vi "TDOanalysis.vi"() -> ()   [LabVIEW 2021]
uses:
  ark_all/arkady-arxiv/oldTDOanalysis/Data window.ctl
  ark_all/arkady-arxiv/agregator -- action.ctl
  ark_all/arkady-arxiv/interpolation state - real.ctl
  ark_all/arkady-arxiv/filename-action.ctl
  <vilib>/Analysis/4window.llb/Hanning Window (DBL).vi
  <vilib>/Analysis/4window.llb/Blackman Window (DBL).vi
  <vilib>/Analysis/baseanly.llb/Mean (DBL).vi
  <vilib>/Analysis/8numeric.llb/1D Numeric Integration.vi
  ark_all/arkady-arxiv/linear interpolation - real -- V2.vi
  <vilib>/Analysis/4window.llb/AllCosWindow (DBL).vi
  <vilib>/Analysis/baseanly.llb/A x B.vi
  <vilib>/Analysis/baseanly.llb/Real A x B.vi
  ark_all/arkady-arxiv/Q -- check range -- i -- real.vi
  ark_all/arkady-arxiv/line -- complex.vi
  ark_all/arkady-arxiv/Q -- check range -- i -- integer.vi
  ark_all/arkady-arxiv/Q - not nan -- real.vi
  ark_all/arkady-arxiv/Q - not nan -- integer.vi
  <vilib>/measure/matone.llb/Extract Single Tone Information 1 Chan.vi
  <vilib>/Waveform/WDTOps.llb/WDT Number of Waveform Samples DBL.vi
  <vilib>/Analysis/Matrix/Numeric/Conversions/Array To Matrix.vi
  <vilib>/Analysis/Matrix/Numeric/Conversions/Array To Matrix - RA2.vi
  <vilib>/Analysis/baseanly.llb/Inverse Matrix.vi
  <vilib>/Analysis/baseanly.llb/Real Inverse Matrix.vi
  <vilib>/Utility/file.llb/Write Delimited Spreadsheet (string).vi
  <vilib>/Utility/file.llb/Write Delimited Spreadsheet (DBL).vi
  <vilib>/Analysis/NI_AALPro.lvlib
  <vilib>/measure/NI_MAPro.lvlib
  <vilib>/Analysis/NI_AALBase.lvlib
  <vilib>/Analysis/NI_AAL_SigProc.lvlib
panel:
  in  "Tab Control":enum32{"Page 1", "Page 2", "Page 3"}(tab)
  in  "gamma window (sec)":dbl=0.0001 format="%#_6p"
  out "Gamma vs. Field":cluster{dbl[], dbl[]}(graph)
  out "Apmlitude or Pwr. vs. Field":cluster{dbl[], dbl[]}(graph)
  out "Frequency vs. Field":cluster{dbl[], dbl[]}(graph)
  out "Frequency vs. time":waveform(dbl)(graph)={"t0"=timestamp(-0.00999989999999995 s since 1904-01-01), "dt"=2e-05, "Y"=array[6499 elements]}
  out "Progress":dbl(slide)=1.0018766168281668 scale=0.0..1.0
  out "first line":string[](array[string])=["003_041224_time 003_041224_field 003_041224_freq 003_041224_amp 003_041224_gamma "]
  in  "remove file prefix":string="p_c3_"
  in  "?":enum32{"TDO Analysis Settings", "Page 2"}(tab)
  in  "Power spctr. threshold":dbl=0.0001 format="%.4f"
  in  "Freq. threshold":dbl=30000.0
  in  "window width (s)":dbl=0.0003 format="%#_6p"
  in  "window step (s)":dbl=2e-05 format="%#_6p"
  in  "detection method":T1(ring)
  in  "fit width":i32=9 min=3
  in  "window type":enum16{"Hanning", "Box", "Blackman"}(ring)
  in  "Input File":path=path "/Users/arkadyshekhter/Library/CloudStorage/Dropbox/shared_KimValBra/Apr2024— UTe2/041224/p_c3_003_041224.tdms"
  out "Ampl vs. time":waveform(dbl)(graph)={"t0"=timestamp(-0.00999989999999995 s since 1904-01-01), "dt"=2e-05, "Y"=array[6499 elements]}
  in  "add file suffix":string="_tdo_"
  in  "ovewrite file?":bool=TRUE
  in  "?":enum32{"data settings", "Field  Settings"}(tab)
  in  "Data channels (1st - Field, 2nd - TDO)":T2={"Start"=0, "Length"=10000, "Other frmt channel numbers"=[0], "TDMS Channel names"=["Field", "Vpick"], "TDMS Group name"="p"}
  in  "Data File Type":T3(ring)
  in  "Bdot Calibration Factor":dbl=3794.0
  out "B dot offset":dbl=-3.6804060216009077e-06 format="%.6f"
  in  "Length for Bdot offset, s":dbl=0.009 format="%#_6p"
  in  "Input field format":enum16{"Bdot", "B"}(ring)=enum."B"
  in  "Field correction":dbl=1.0
  out "Array":bool[](array[boolean])
  in  "upper limit":dbl
  in  "lower limit":dbl
  in  "Low-pass filter":T4={"Clip IIR filter ramps, in 1/Tc units"=1.0, "Two-pass & flip"=TRUE, "IIR filter specifications"={"Topology"=enum."Off", "Type"=enum."Lowpass", "Order"=1, "Lower Fc"=1e-06, "Upper Fc"=0.0, "PB Ripple"=1.0, "SB Attenuation"=60.0}} {"IIR filter specifications"."PB Ripple" format="%0.2f"; "IIR filter specifications"."Lower Fc" format="%0.2p"; "IIR filter specifications"."SB Attenuation" format="%0.2f"; "IIR filter specifications"."Upper Fc" format="%0.2p"}
  in  "error in":errorcluster
  out "Amplitude vs. Field (PWR peak)":cluster{dbl[], "Filtered X":dbl[]}(graph)
  out "size(s)":i32=6499
  in  "# of threads":i32=4
  out "Field profile":waveform(dbl)(graph)={"t0"=timestamp(-0.00999989999999995 s since 1904-01-01), "dt"=2e-05, "Y"=array[6468 elements]}
  in  "End, s":dbl=nan format="%.6f"
  in  "Start, s":dbl=nan format="%.6f"
  # "Basic NHMFL TDO routine\nv. 0.5       F. F. Balakirev\n\nmessed with by Arkady!"
  # "Background file is either an ASCII *.dat file produced by TDO earlier\nor *.fit file containing single column of polynomial fit coeficients.\n1st row in fit file is a text header, which is ingnored. Result is saved in a \n\"*diff.dat\" file in the output folder\nExample \"PDO1.fit\": \n\nFit y=A_i*x^i, starting with A_0\n3.25637E7\n2132.56863\n-12.60591\n-2.01013\n-0.04452\n-3.23119E-4"
  # "OR"
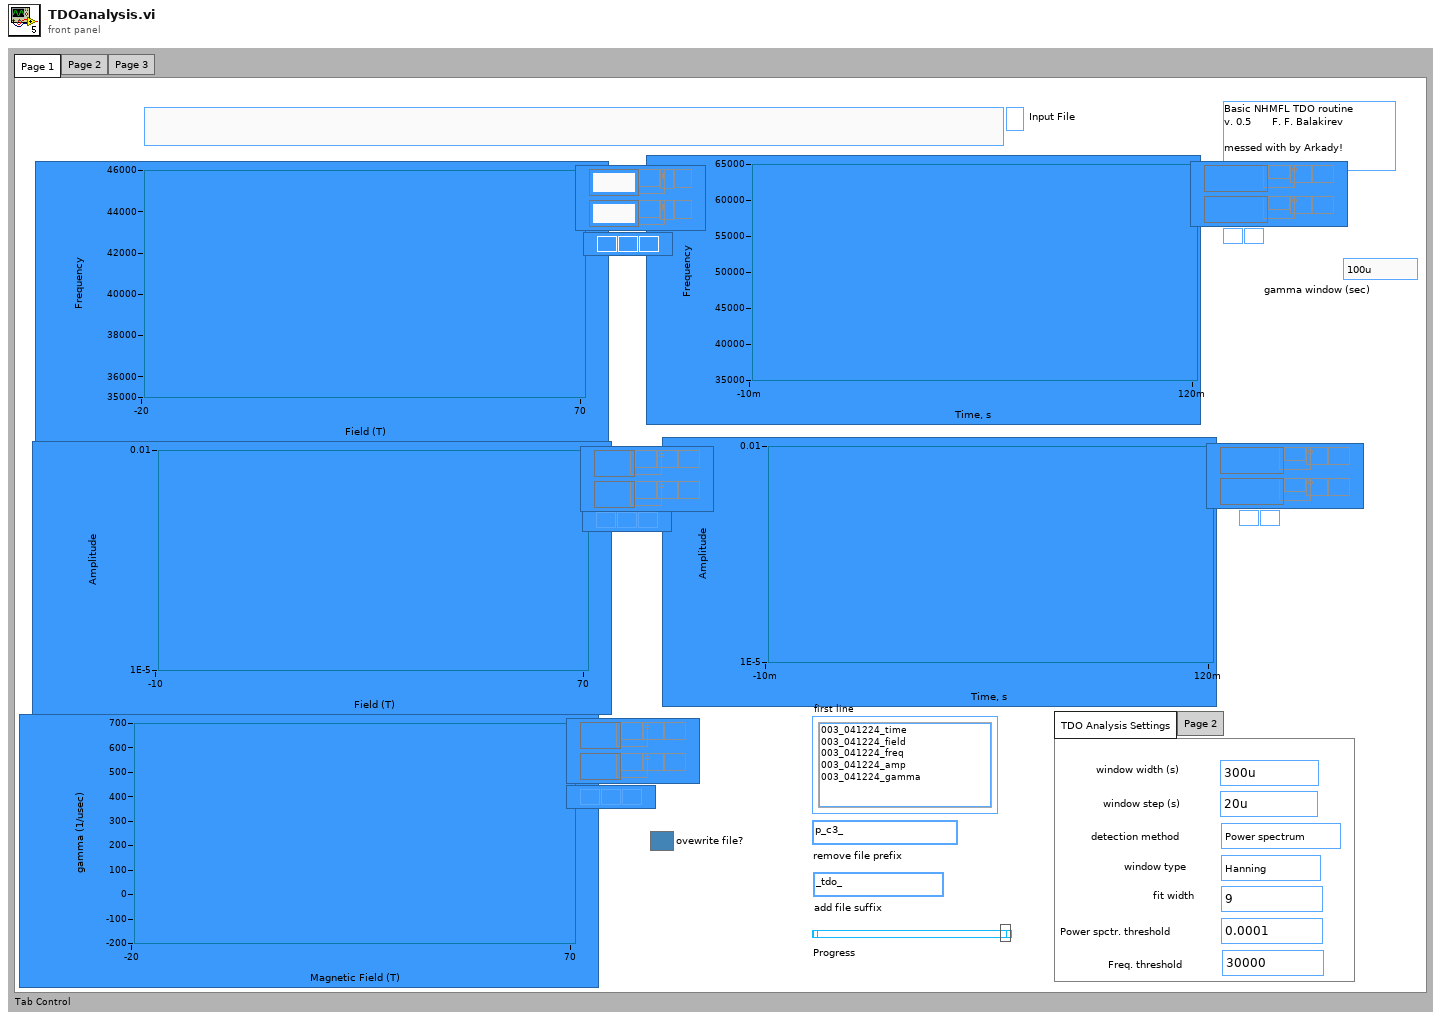
[diagram p1: front panel]
types:
  T1 = enum16{"Power spectrum", "Tone detection", "Peak-to-peak fit"}
  T2 = cluster{"Start":i64, "Length":i32, "Other frmt channel numbers":i64[], "TDMS Channel names":string[], "TDMS Group name":string}
  T3 = enum16{"TDMS file", "Tektronics ISF", "BinF file", "ASCII File", "BinH File", "BinW File", "BINARY File"}
  T4 = cluster{"Clip IIR filter ramps, in 1/Tc units":dbl, "Two-pass & flip":bool, "IIR filter specifications":cluster{"Topology":enum16{"Off", "Butterworth", "Chebyshev", "Inverse Chebyshev", "Elliptic", "Bessel"}, "Type":enum16{"Lowpass", "Highpass", "Bandpass", "Bandstop"}, "Order":i32, "Lower Fc":dbl, "Upper Fc":dbl, "PB Ripple":dbl, "SB Attenuation":dbl}}
  T5 = typedef "filename-action.ctl" = enum16{"rewrite", "parse", "force pattern", "uniquenum", "get T", "get B", "get ind", "get deg", "get name", "get folder", "get extension", "get basename", "get side", "get setof", "getID", "getIDStock", "remove prefix"}
  T6 = typedef "interpolation state - real.ctl" = cluster{"Array ":dbl[], "actual size":i32, "requested size":i32}
  T7 = typedef "agregator -- action.ctl" = enum16{"append", "interpolate", "empty!", "force", "init", "scale", "read last"}
  T8 = enum16{"Off", "Butterworth", "Chebyshev", "Inverse Chebyshev", "Elliptic", "Bessel"}
  T9 = cluster{"Start":i64, "Length":i64, "Channel numbers":i64[], "Channel names":string[], "Group name":string}
  T10 = typedef "Data window.ctl" = cluster{"Start":i64, "Length":i64, "Channel numbers":i64[], "Channel name":string, "Group name":string}
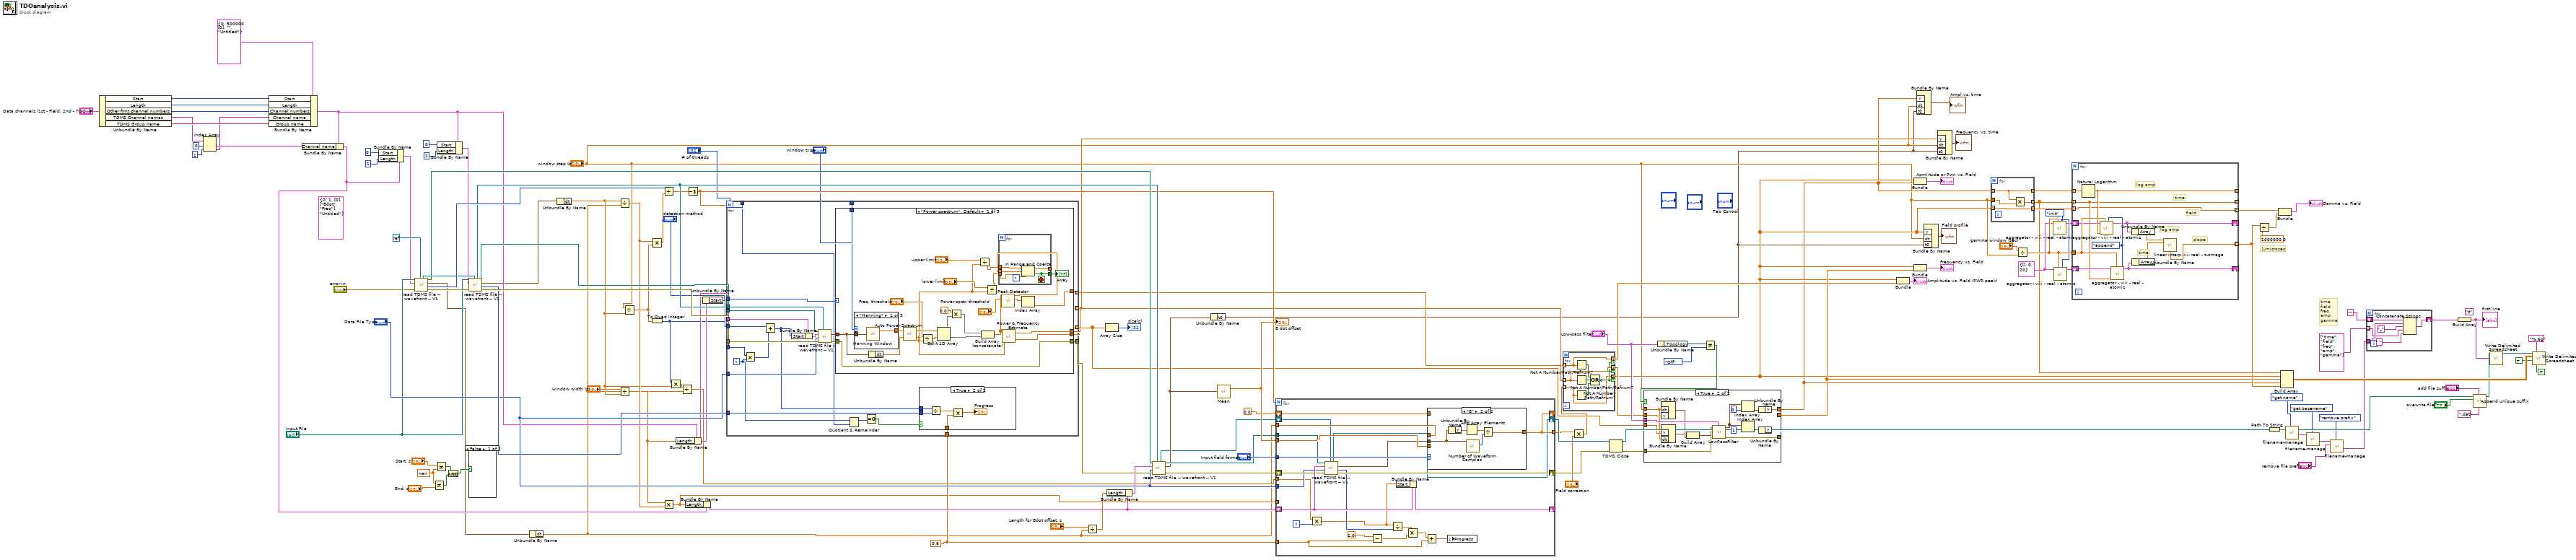
[diagram p0: block diagram]
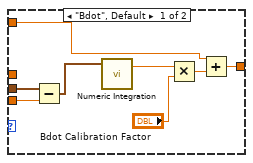
[diagram p2: hidden frame]
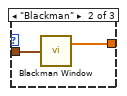
[diagram p5: hidden frame]
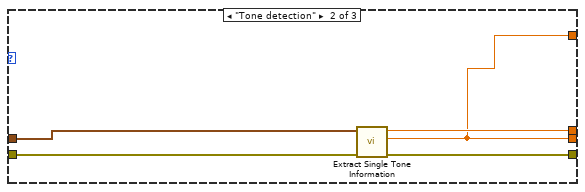
[diagram p7: hidden frame]
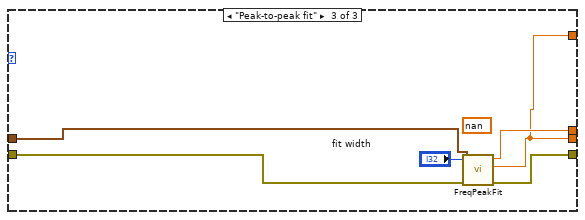
[diagram p8: hidden frame]
diagram:
  (unwired) "\t"
  w33 = T6 {"Array "=[], "actual size"=0, "requested size"=20} ("state IN")
  w38 = agregator_--_action."init" ("aggregator action")
  w68 = 0.6 ("y")
  (unwired) T9 {"Start"=0, "Length"=1, "Channel numbers"=[0], "Channel names"=["Bdot", "Freq"], "Group name"="Untitled"} ("Data window")
  w112 = nan
  # "1/microsec"
  # "time \nfield\nfreq\namp\ngamma"
  n1 = Unbundle By Name("Data channels (1st - Field, 2nd - TDO)") -> ("Start"=w118:i64, "Length"=w121:i32, "Other frmt channel numbers"=w120:i64[], "TDMS Channel names"=w100:string[], "TDMS Group name"=w119:string)
  n2 = Index Array(array=w100, index #1=0 ("index"), index #2=1 ("index")) -> (element #1=w117:string, element #2=w104:string)
  n3 = Bundle By Name(cluster=T10 {"Start"=0, "Length"=500000, "Channel numbers"=[0], "Channel name"="", "Group name"="Untitled"} ("Data window"), "Start"=w118, "Length"=w121, "Channel numbers"=w120, "Channel name"=w104, "Group name"=w119) -> (w102:T10)
  n4 = Bundle By Name(cluster=w102, "Channel name"=w117) -> (w116:T10)
  n5 = Bundle By Name(cluster=w116, "Start"=i64 0, "Length"=i64 1) -> (w97:T10)
  n6 = call "read TDMS file -- wavefront -- V1.vi"("tdms file in"=refnum<k0> refnum, "error in"="error in", "Data window"=w97, "Input file path"="Input File") -> ("error out"=w132:errorcluster, "1st channel length"=w126:u64, "Data out"=w99:waveform(dbl), "Actual input file path"=w128:path, "tdms file out"=w106:refnum<k34>)  [unwired: 3 in]
  n7 = Not Equal?(x=w112, y="End, s") -> (x != y?=w109:bool)
  n8 = Not Equal?(x="Start, s", y=w112) -> (x != y?=w110:bool)
  n9 = Bundle By Name(cluster=w102, "Start"=i64 0, "Length"=i64 1) -> (w96:T10)
  n10 = And(x=w110, y=w109) -> (x .and. y?=w108:bool)
  n11 = case shown="False" w108 {
    frame False {
    }
    frame True {
    }
  }
  n12 = call "read TDMS file -- wavefront -- V1.vi"("tdms file in"=w106, "error in"=w132, "Data window"=w96, "Input file path"="Input File") -> ("error out"=w129:errorcluster, "1st channel length"=w125:u64, "Data out"=w98:waveform(dbl), "Actual input file path"=w131:path, "tdms file out"=w107:refnum<k34>)  [unwired: 3 in]
  n13 = Unbundle By Name(w99) -> ("dt"=w31:dbl)
  n14 = Unbundle By Name(w98) -> ("dt"=w32:dbl)
  n15 = Divide(x=w32, y=w31) -> (x/y=w62:dbl)
  n16 = Divide(x="window width (s)", y=w32) -> (x/y=w57:dbl)
  n17 = Divide(x="window step (s)", y=w32) -> (x/y=w88:dbl)
  n18 = Multiply(x=w62, y=w88) -> (x*y=w76:dbl)
  n19 = To Quad Integer(1:w88) -> (0:w56:i64)
  n20 = Divide(x=w126, y=w76) -> (x/y=w95:dbl)
  n21 = Multiply(x=w57, y=w62) -> (x*y=w58:dbl)
  n22 = Multiply(x=w56, y=w32) -> (x*y=w55:dbl)
  n23 = Bundle By Name(cluster=w102, "Length"=w57) -> (w61:T10)
  n24 = Divide(x=w55, y=w31) -> (x/y=w54:dbl)
  n25 = Bundle By Name(cluster=w116, "Length"=w58) -> (w77:T10)
  n26 = Decrement(x=w95) -> (x-1=w69:dbl)
  n27 = Unbundle By Name(w61) -> ("Start"=w60:i64)
  n28 = for {
    N: w69 -> [_]
    tunnel: [w152] -> w51 mode=indexing
    tunnel: [w157] -> w52 mode=indexing
    tunnel: [w156] -> w50 mode=indexing
    tunnel: "Data File Type" -> [w153]
    tunnel: w131 -> [w154]
    tunnel: w56 -> [w145]
    tunnel: "detection method" -> [w151]
    tunnel: w125 -> [w150]
    tunnel: w68 -> [w147]
    tunnel: w61 -> [w144]
    tunnel: w60 -> [w143]
    tunnel: w129 -> [w155]
    tunnel: [w149] -> w71
    tunnel: "window type" -> [w141]
    tunnel: w107 -> [w135]
    tunnel: "# of threads" -> [w134]
    i -> [w138]
    n29 = Multiply(x=w145, y=w138) -> (x*y=w139:i64)
    n30 = Add(x=w143, y=w139) -> (x+y=w140:i64)
    n31 = Bundle By Name(cluster=w144, "Start"=w140) -> (w142:T10)
    n32 = call "read TDMS file -- wavefront -- V1.vi"("tdms file in"=w135, "error in"=w155, "Data File Type"=w153, "Data window"=w142, "Input file path"=w154) -> ("error out"=w148:errorcluster, "Data out"=w146:waveform(dbl))  [unwired: 2 in, 3 out]
    n33 = case shown="\"Power spectrum\", Default" w151 {
      tunnel: [w186 w198 w203] -> w157
      tunnel: [w167 w198 w203] -> w156
      tunnel: w146 -> [w185 w201 w208]
      tunnel: [w174 w202 w207] -> w152
      tunnel: w148 -> [w176 w200 w205]
      tunnel: [w176 w199 w204] -> w149
      tunnel: w141 -> [w175 _ _]
      frame "Power spectrum", Default {
        n34 = case shown="\"Hanning\"" w175 {
          tunnel: [w194 w196 w197] -> w187
          tunnel: w185 -> [w193 w195 w197]
          frame "Hanning" {
            n35 = call-poly <vilib>:"Hanning Window.vi"("X"=w193) -> ("Windowed X"=w194:dbl[])  [unwired: 1 out]
          }
          frame "Blackman" {
            n36 = call-poly <vilib>:"Blackman Window.vi"("X"=w195) -> ("Windowed X"=w196:dbl[])  [unwired: 1 out]
          }
          frame "Box" {
          }
        }
        n37 = Unbundle By Name(w185) -> ("dt"=w184:dbl)
        n38 = call <vilib>:"Auto Power Spectrum.vi"("dt"=w184, "Signal (V)"=w187) -> ("df"=w171:dbl, "Power Spectrum (V^2 rms)"=w182:dbl[])
        n39 = Divide(x="Freq. threshold", y=w171) -> (x/y=w181:dbl)
        n40 = Split 1D Array(array=w182, index=w181) -> (first subarray=w178:dbl[], second subarray=w180:dbl[])
        n41 = Multiply(x=0.0 ("element"), y=w178) -> (x*y=w177:dbl[])
        n42 = Divide(x="upper limit", y=w171) -> (x/y=w169:dbl)
        n43 = Build Array (concatenate)(w177, w180) -> (w166:dbl[])
        n44 = Divide(x="lower limit", y=w171) -> (x/y=w172:dbl)
        n45 = call <vilib>:"Peak Detector.vi"("threshold"="Power spctr. threshold", "X"=w166) -> ("Amplitudes"=w163:dbl[], "Locations"=w164:dbl[])  [unwired: 5 in, 3 out]
        n46 = for {
          tunnel: w164 -> [w192] mode=indexing
          tunnel: w169 -> [w191]
          tunnel: w172 -> [w190]
          tunnel: [w189] -> _
          tunnel: [w188] -> w168 mode=indexing
          stop <- w188 stop-if-true
          n47 = In Range and Coerce(upper limit=w191, x=w192, lower limit=w190) -> (coerced(x)=w189:dbl, In Range?=w188:bool)
        }
        "Array" <- w168
        n48 = call <vilib>:"Power & Frequency Estimate.vi"("df"=w171, "Power Spectrum (V^2 rms)"=w166) -> ("est power peak"=w186:dbl, "est frequency peak"=w174:dbl)  [unwired: 3 in, 1 out]
        n49 = Index Array(array=w163) -> (element=w167:dbl)  [unwired: 1 in]
      }
      frame "Tone detection" {
        n50 = call-poly <vilib>:"Extract Single Tone Information.vi"("error in (no error)"=w200, "time signal in"=w201) -> ("error out"=w199:errorcluster, "detected amplitude"=w198:dbl, "detected frequency"=w202:dbl)  [unwired: 2 in, 5 out]
      }
      frame "Peak-to-peak fit" {
        (unwired) nan
        n51 = call "FreqPeakFit.vi"("error in (no error)"=w205, "Peak fit width"="fit width", "Waveform"=w208) -> ("error out"=w204:errorcluster, "Amplitude"=w203:dbl, "PeakFreqOut"=w207:dbl)  [unwired: 4 out]
      }
    }
    n52 = Quotient & Remainder(x=w138, y=w134) -> (x-y*floor(x/y)=w137:i32)  [unwired: 1 out]
    n53 = Equal To 0?(x=w137) -> (x = 0?=w136:bool)
    n54 = case shown="True" w136 {
      tunnel: w150 -> [_ w162]
      tunnel: w147 -> [_ w159]
      tunnel: w140 -> [_ w158]
      frame False {
      }
      frame True {
        n55 = Divide(x=w158, y=w162) -> (x/y=w161:dbl)
        n56 = Multiply(x=w161, y=w159) -> (x*y=→"Progress":dbl)
      }
    }
  }
  n57 = Divide(x="Length for Bdot offset, s", y=w31) -> (x/y=w79:dbl)
  n58 = Array Size(array=w52) -> (size(s)=→"size(s)":i32)
  n59 = Bundle By Name(cluster=w77, "Length"=w79) -> (w67:T10)
  n60 = call "read TDMS file -- wavefront -- V1.vi"("tdms file in"=w107, "error in"=w71, "Data File Type"="Data File Type", "Data window"=w67, "Input file path"=w128) -> ("error out"=w70:errorcluster, "Data out"=w66:waveform(dbl), "Actual input file path"=w72:path, "tdms file out"=w65:refnum<k34>)  [unwired: 2 in, 1 out]
  n61 = Unbundle By Name(w66) -> ("t0"=w4:timestamp)
  n62 = call-poly <vilib>:"Mean.vi"("X"=w66) -> ("mean"=w74:dbl)  [unwired: 1 out]
  "B dot offset" <- w74
  n63 = for {
    N: w69 -> [_]
    shift-right: [w229] -> w78
    shift-left: w70 -> [w230]
    shift-right: [w232] -> _
    shift-left: w77 -> [w231]
    tunnel: w54 -> [w211]
    tunnel: "Input field format" -> [w228]
    tunnel: w74 -> [w227]
    shift-right: [w226] -> _
    shift-left: 0.0 -> [w225]
    tunnel: [w226] -> w46 mode=indexing
    tunnel: w31 -> [w224]
    tunnel: w72 -> [w223]
    tunnel: w68 -> [w209]
    shift-right: [w214] -> w63
    shift-left: w65 -> [w215]
    tunnel: "Data File Type" -> [w213]
    tunnel: w58 -> [_]
    i -> [w212]
    n64 = Multiply(x=w211, y=w212) -> (x*y=w210:dbl)
    n65 = call "read TDMS file -- wavefront -- V1.vi"("tdms file in"=w215, "error in"=w230, "Data File Type"=w213, "Data window"=w231, "Input file path"=w223) -> ("error out"=w229:errorcluster, "1st channel length"=w221:u64, "Data out"=w216:waveform(dbl), "tdms file out"=w214:refnum<k34>)  [unwired: 2 in, 1 out]
    n66 = Subtract(x=1.0, y=w209) -> (x-y=w219:dbl)
    n67 = Divide(x=w210, y=w221) -> (x/y=w222:dbl)
    n68 = Bundle By Name(cluster=w231, "Start"=w210) -> (w232:T10)
    n69 = Multiply(x=w222, y=w219) -> (x*y=w217:dbl)
    n70 = Add(x=w217, y=w209) -> (x+y=w218:dbl)
    n71 = case shown="\"B\"" w228 {
      tunnel: w225 -> [w240 _]
      tunnel: [w238 w242] -> w226
      tunnel: w227 -> [w236 _]
      tunnel: w224 -> [_ _]
      tunnel: w216 -> [w234 w241]
      frame "Bdot", Default {
        n72 = Subtract(x=w234, y=w236) -> (x-y=w237:waveform(dbl))
        n73 = call-poly <vilib>:"Numeric Integration.vi"("Input Array"=w237) -> ("result"=w235:dbl)  [unwired: 2 in, 1 out]
        n74 = Multiply(x=w235, y="Bdot Calibration Factor") -> (x*y=w239:dbl)
        n75 = Add(x=w240, y=w239) -> (x+y=w238:dbl)
      }
      frame "B" {
        n76 = Unbundle By Name(w241) -> ("Y"=w245:dbl[])
        n77 = Add Array Elements(numeric array=w245) -> (sum=w243:dbl)
        n78 = call-poly <vilib>:"Number of Waveform Samples.vi"("waveform in"=w241) -> ("number of samples"=w244:i32)  [unwired: 1 in, 9 out]
        n79 = Divide(x=w243, y=w244) -> (x/y=w242:dbl)
      }
    }
    n80 = local write "Progress"(w218) -> ()
  }
  n81 = Multiply(x=w46, y="Field correction") -> (x*y=w44:dbl[])
  n82 = for {
    tunnel: w51 -> [w251] mode=indexing
    tunnel: w44 -> [w250] mode=indexing
    tunnel: w50 -> [w252] mode=indexing
    tunnel: [w252] -> w47 mode=indexing if=w246
    tunnel: [w251] -> w48 mode=indexing if=w246
    tunnel: [w250] -> w42 mode=indexing if=w246
    n83 = Not A Number/Path/Refnum?(number/path/refnum=w252) -> (NaN/Path/Refnum?=w249:bool)
    n84 = Not A Number/Path/Refnum?(number/path/refnum=w251) -> (NaN/Path/Refnum?=w248:bool)
    n85 = Not A Number/Path/Refnum?(number/path/refnum=w250) -> (NaN/Path/Refnum?=w247:bool)
    n86 = Compound Arithmetic op=OR(w249, w248, w247) -> (invert w246:bool)
  }
  n87 = TDMS Close(8:w78, 11:w63) -> (0:w64:errorcluster, 3:w20:path)
  n88 = Unbundle By Name("Low-pass filter") -> ("IIR filter specifications.Topology"=w85:T8)
  n89 = Not Equal?(x=w85, y=T8."Off" ("IIR filter specifications.Topology")) -> (x != y?=w84:bool)
  n90 = case shown="True" w84 {
    tunnel: w64 -> [w255 w271]
    tunnel: [w255 w270] -> _
    tunnel: "Low-pass filter" -> [_ w269]
    tunnel: w52 -> [w254 w267]
    tunnel: w48 -> [w253 w268]
    tunnel: "window step (s)" -> [_ w256]
    tunnel: [w253 w258] -> w49
    tunnel: [w254 w257] -> w6
    frame False {
    }
    frame True {
      n91 = Bundle By Name("dt"=w256, "Y"=w268) -> (w265:waveform(dbl))  [unwired: 1 out]
      n92 = Bundle By Name("Y"=w267, "dt"=w256) -> (w266:waveform(dbl))  [unwired: 1 out]
      n93 = Build Array(w266, w265) -> (w264:waveform(dbl)[])
      n94 = call "LowPassFilter.vi"("Low-pass filter"=w269, "error in (no error)"=w271, "signal(s) in"=w264) -> ("error out"=w270:errorcluster, "signal(s) out"=w263:waveform(dbl)[])  [unwired: 2 in, 5 out]
      n95 = Index Array(array=w263, index=0) -> (element=w260:waveform(dbl))
      n96 = Index Array(array=w263, index=1) -> (element=w259:waveform(dbl))
      n97 = Unbundle By Name(w260) -> ("Y"=w257:dbl[])
      n98 = Unbundle By Name(w259) -> ("Y"=w258:dbl[])
    }
  }
  n99 = Bundle(w42, w47) -> (→"Amplitude vs. Field (PWR peak)":cluster{dbl[], dbl[]})  [unwired: 1 out]
  n100 = Bundle(w42, "Y"=w6) -> (→"Apmlitude or Pwr. vs. Field":cluster{dbl[], "Y":dbl[]})  [unwired: 1 out]
  n101 = Bundle(w42, "Y"=w49) -> (→"Frequency vs. Field":cluster{dbl[], "Y":dbl[]})  [unwired: 1 out]
  n102 = Bundle By Name("Y"=w6, "dt"="window step (s)", "t0"=w4) -> (→"Ampl vs. time":waveform(dbl))  [unwired: 1 out]
  n103 = Bundle By Name("Y"=w42, "dt"="window step (s)", "t0"=w4) -> (→"Field profile":waveform(dbl))  [unwired: 1 out]
  n104 = Bundle By Name("Y"=w51, "dt"="window step (s)", "t0"=w4) -> (→"Frequency vs. time":waveform(dbl))  [unwired: 1 out]
  n105 = for {
    tunnel: w6 -> [w273] mode=indexing
    tunnel: "window step (s)" -> [w275]
    tunnel: [w274] -> w30 mode=indexing
    tunnel: [w273] -> w40 mode=indexing
    tunnel: [w272] -> w36 mode=indexing
    tunnel: w42 -> [w272] mode=indexing
    n106 = Multiply(x=w273, y=w275) -> (x*y=w274:dbl)
  }
  n107 = Divide(x="gamma window (sec)", y="window step (s)") -> (x/y=w39:dbl)
  n108 = call "aggregator - viii - real - atomic.vi"("aggregator action"=w38, "requested size"=w39, "state IN"=w33) -> ("state OUT"=w37:T6)  [unwired: 5 in, 3 out]
  n109 = call "aggregator - viii - real - atomic.vi"("aggregator action"=w38, "requested size"=w39, "state IN"=w33) -> ("state OUT"=w41:T6)  [unwired: 5 in, 3 out]
  n110 = for {
    shift-right: [w282] -> _
    shift-left: w41 -> [w288]
    tunnel: w39 -> [w285]
    tunnel: w40 -> [w287] mode=indexing
    tunnel: w30 -> [w277] mode=indexing
    shift-right: [w283] -> _
    shift-left: w37 -> [w284]
    tunnel: [w279] -> w9 mode=indexing
    tunnel: [w278] -> _ mode=indexing
    tunnel: [w277] -> _ mode=indexing
    tunnel: w36 -> [w276] mode=indexing
    tunnel: [w276] -> w35 mode=indexing
    w286 = agregator_--_action."append" ("aggregator action")
    # "field"
    # "slope"
    # "time"
    # "log amp"
    # "log amp"
    # "time"
    n111 = Natural Logarithm(1:w287) -> (0:w278:dbl)
    n112 = call "aggregator - viii - real - atomic.vi"("aggregator action"=w286, "requested size"=w285, "number"=w278, "state IN"=w284) -> ("state OUT"=w283:T6)  [unwired: 4 in, 3 out]
    n113 = call "aggregator - viii - real - atomic.vi"("aggregator action"=w286, "requested size"=w285, "number"=w277, "state IN"=w288) -> ("state OUT"=w282:T6)  [unwired: 4 in, 3 out]
    n114 = Unbundle By Name(w283) -> ("Array"=w280:dbl[])
    n115 = Unbundle By Name(w282) -> ("Array"=w281:dbl[])
    n116 = call "linear interp iiii- real - z-omega.vi"("z"=w280, "omega"=w281) -> ("slope"=w279:dbl)  [unwired: 4 in, 9 out]
  }
  n117 = Divide(x=w9, y=1000000.0) -> (x/y=w7:dbl[])
  n118 = Path To String(path=w20) -> (string=w18:string)
  n119 = Bundle(w35, w7) -> (→"Gamma vs. Field":cluster{dbl[], dbl[]})  [unwired: 1 out]
  n120 = Build Array(w30, w42, w49, w6, w9) -> (w93:dbl[][])
  n121 = call "filename-manage.vi"("filename-action"=filename-action."get name", "file name IN"=w18) -> ("string OUT"=w17:string)  [unwired: 7 in, 2 out]
  n122 = call "filename-manage.vi"("filename-action"=filename-action."get basename", "file name IN"=w17) -> ("string OUT"=w15:string)  [unwired: 7 in, 2 out]
  n123 = call "filename-manage.vi"("filename-action"=filename-action."remove prefix", "string IN"="remove file prefix", "file name IN"=w15) -> ("string OUT"=w12:string)  [unwired: 6 in, 2 out]
  n124 = for {
    tunnel: string[] ["time", "field", "freq", "amp", "gamma"] -> [w290] mode=indexing
    shift-right: [w293] -> w10
    shift-left: "" ("format (%.3f)") -> [w294]
    tunnel: w12 -> [w292]
    n125 = Concatenate Strings(w294, w292, "_", w290, " ") -> (w293:string)
  }
  n126 = Build Array(w10) -> (w22:string[])
  "first line" <- w22
  n127 = call "Append unique suffix.vi"("Extention"=".dat", "Suffix"="add file suffix", "ovewrite ?"="ovewrite file?", "Path"=w20) -> ("Path out"=w23:path)  [unwired: 6 in, 1 out]
  n128 = call-poly <vilib>:"Write Delimited Spreadsheet.vi"("file path (dialog if empty)"=w23, "1D data"=w22) -> ("new file path (Not A Path if cancelled)"=w21:path)  [unwired: 12 in, 1 out]
  n129 = call-poly <vilib>:"Write Delimited Spreadsheet.vi"("file path (dialog if empty)"=w21, "format (%.3f)"="%.6g", "2D data"=w93, "append to file? (new file:F)"=TRUE, "transpose? (no:F)"=TRUE) -> ()  [unwired: 9 in, 2 out]
